vi "Dosing.vi"() -> ()   [LabVIEW 2019]
uses:
  <vilib>/NI/Current Value Table/Type Defs/Single Tag.ctl
  <vilib>/NI/Current Value Table/Type Defs/Data Types.ctl
  <vilib>/NI/STM/TCP/Read Meta Data (TCP Ref).vi
  <vilib>/NI/STM/TCP/Get Connection Reference (TCP).vi
  <vilib>/NI/AMC/Read Termination Message.vi
  <vilib>/NI/AMC/Create Single Message.vi
  <vilib>/NI/AMC/Update Message Routing Info.vi
  <vilib>/NI/STM/TCP/Read Meta Data (TCP Clst).vi
  <vilib>/NI/AMC/Globals.vi
  <vilib>/NI/STM/TCP/Write Message (TCP).vi
  <vilib>/NI/AMC/Send Message.vi
  <vilib>/NI/AMC/AMC.lvlib
  <vilib>/NI/STM/NI STM.lvlib
  <vilib>/NI/Current Value Table/Current Value Table.lvlib
panel:
  in  "Sulfuric Proc 3":dbl=2.0 caption="ml Acid Proc 3" min=0.0 max=5000.0 step=1.0
  in  "Trig Sulfuric Proc 3":bool caption="Trigger Dose"
  in  "Sulfuric Proc 2":dbl=2.0 caption="ml Acid Proc 2" min=0.0 max=5000.0 step=1.0
  in  "Trig Sulfuric Proc 2":bool caption="Trigger Dose"
  in  "Sulfuric Proc 1":dbl=2.0 caption="ml Acid Proc 1" min=0.0 max=5000.0 step=1.0
  in  "Trig Sulfuric Proc1":bool caption="Trigger Dose"
  in  "LEV Proc 3":dbl=2.0 caption="ml Lev Proc 3" min=0.0 max=1000.0 step=1.0
  in  "Trig Level Proc 3":bool caption="Trigger Dose"
  in  "LEV Proc 2":dbl=2.0 caption="ml Lev Proc 2" min=0.0 max=1000.0 step=1.0
  in  "Trig Level Proc 2":bool caption="Trigger Dose"
  in  "LEV Proc 1":dbl=2.0 caption="ml Lev Proc 1" min=0.0 max=1000.0 step=1.0
  in  "Trig Level Proc1":bool caption="Trigger Dose"
  in  "UCON Proc 3":dbl=2.0 caption="ml UCON Proc 3" min=0.0 max=1000.0 step=1.0
  in  "Trig UCON Proc 3":bool caption="Trigger Dose"
  in  "UCON Proc 2":dbl=2.0 caption="ml UCON Proc 2" min=0.0 max=1000.0 step=1.0
  in  "Trig UCON Proc 2":bool caption="Trigger Dose"
  in  "UCON Proc 1":dbl=2.0 caption="ml UCON Proc 1" min=0.0 max=1000.0 step=1.0
  in  "Trig UCON Proc 1":bool caption="Trigger Dose"
  in  "SPS Proc 3":dbl=2.0 caption="ml SPS Proc 3" min=0.0 max=1000.0 step=1.0
  in  "Trig SPS Proc 3":bool caption="Trigger Dose"
  in  "SPS Proc 2":dbl=2.0 caption="ml SPS Proc 2" min=0.0 max=1000.0 step=1.0
  in  "Trig SPS Proc 2":bool caption="Trigger Dose"
  in  "SPS Proc 1":dbl=2.0 caption="ml SPS Proc 1" min=0.0 max=1000.0 step=1.0
  in  "Trig SPS Proc 1":bool caption="Trigger Dose"
  out "Run Enabled":bool
  in  "Dosing":bool
  in  "Mixing Tank":bool
  in  "Process 3":bool
  in  "Process 2":bool
  in  "Process 1":bool
  out "status":string
  in  "Home Btn":bool
  in  "Facilities Btn":bool
  # "SPS"
  # "UCON"
  # "Leveler"
  # "Sulfuric Acid"
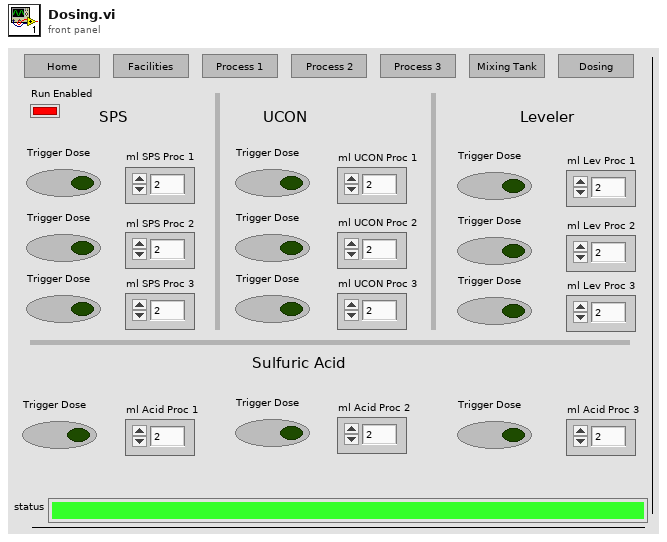
[diagram p1: front panel]
types:
  T1 = typedef "Current Value Table.lvlib/Single Tag.ctl" = cluster{"Data Type":T2, "Name":string, "Value":string, "Description":string}
  T2 = typedef "Current Value Table.lvlib/Data Types.ctl" = enum16{"Double", "Single", "I64", "I32", "I16", "I8", "U64", "U32", "U16", "U8", "String", "Boolean", "Array of U8", "Array of U16", "Array of U32", "Array of U64", "Array of I64", "Array of I32", "Array of I16", "Array of I8", "Array of Double", "Array of Single", "Array of Boolean", "Array of String"}
  T3 = typedef "AMC.lvlib/Message Queue.ctl" = refnum<queue>
  T4 = typedef "NI STM.lvlib/TCP Connection Info.ctl" = cluster{"connection ID":refnum<k5>, "meta data":T5[]}
  T5 = typedef "NI STM.lvlib/MetaDataElement.ctl" = string
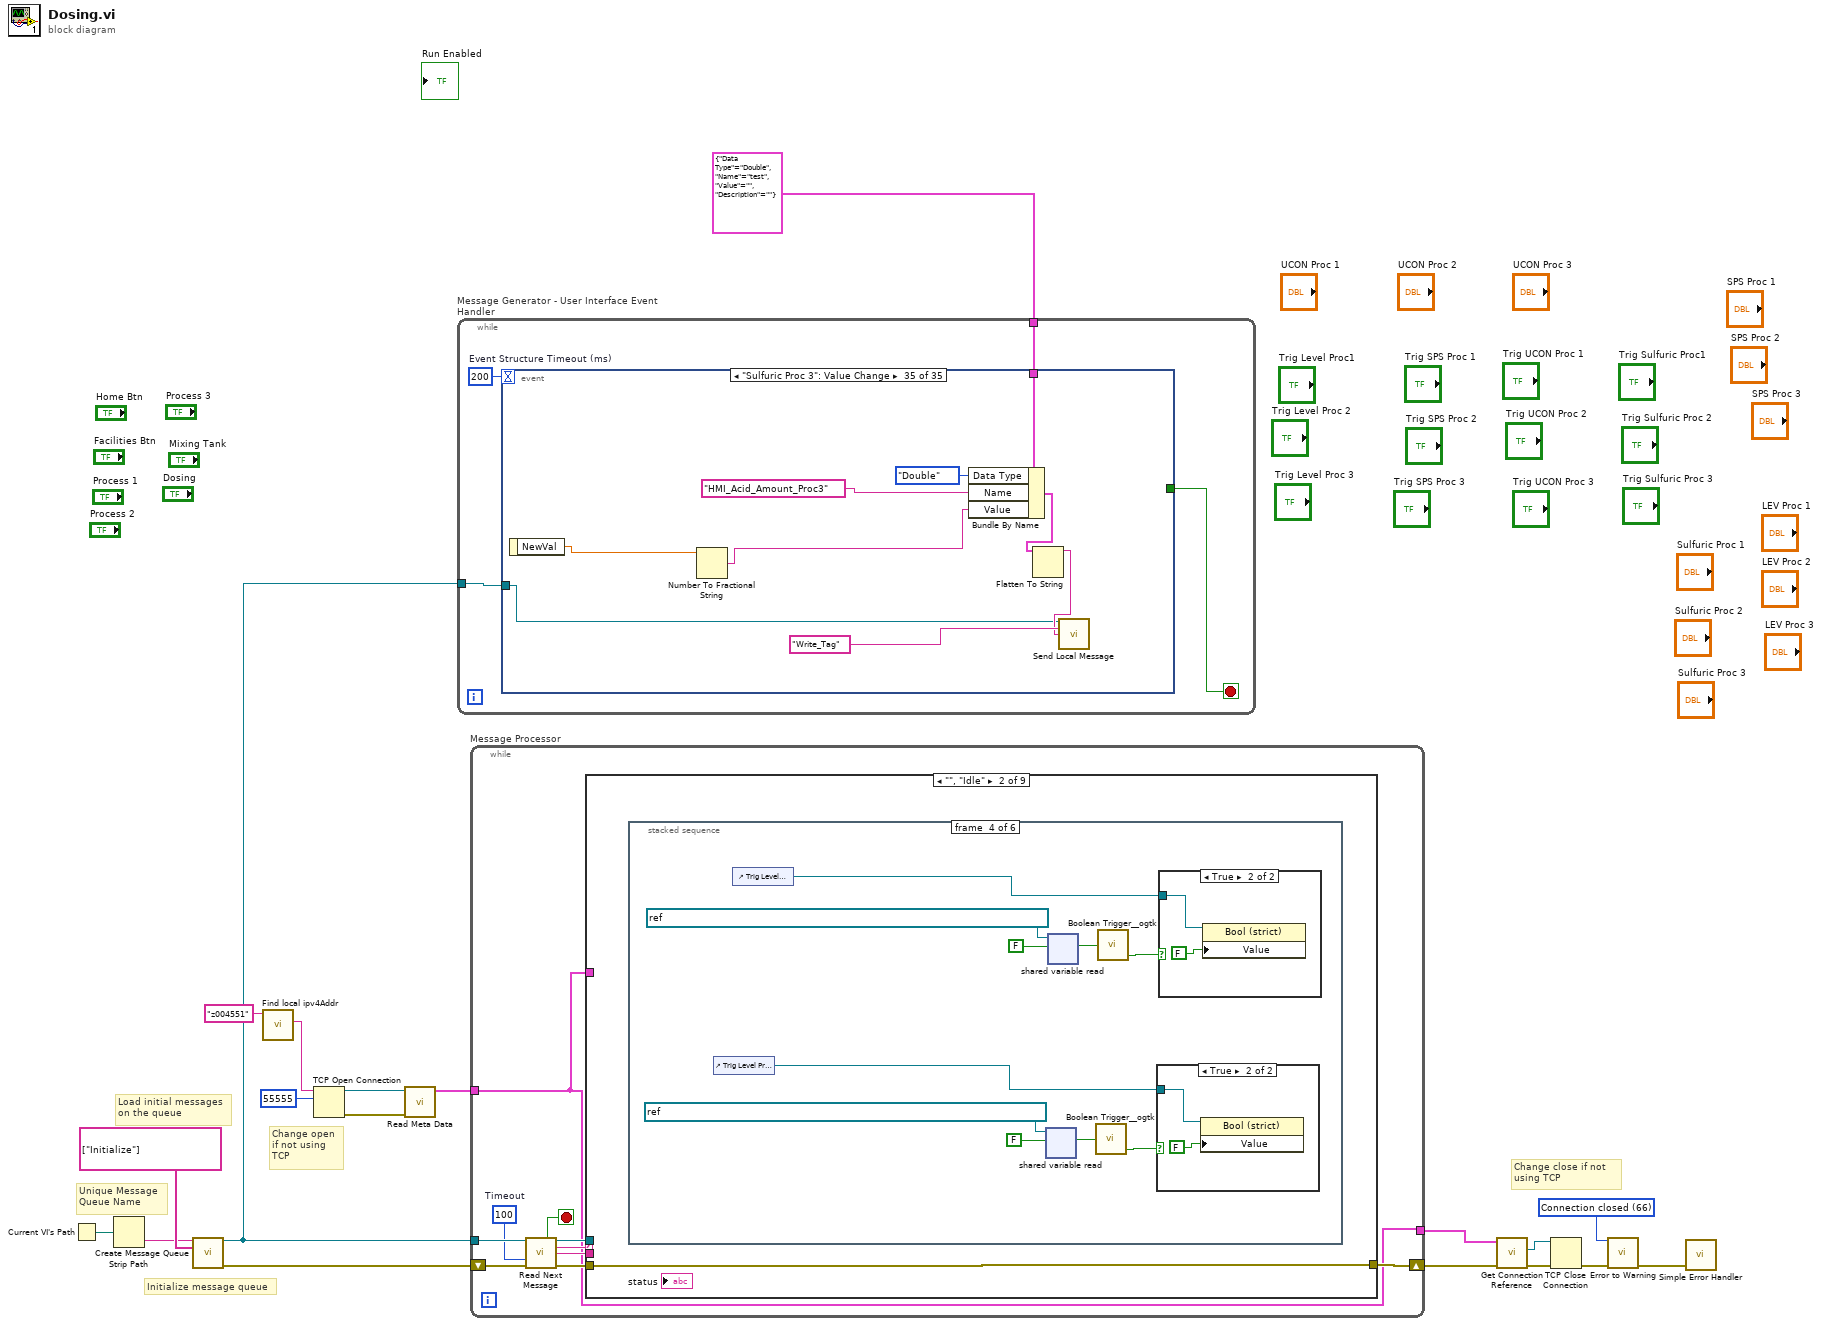
[diagram p0: block diagram]
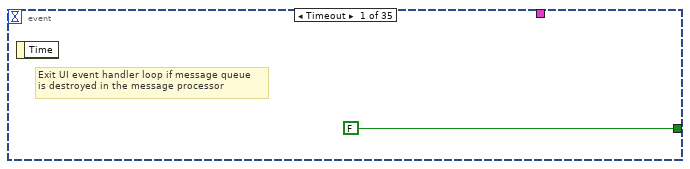
[diagram p2: hidden frame]
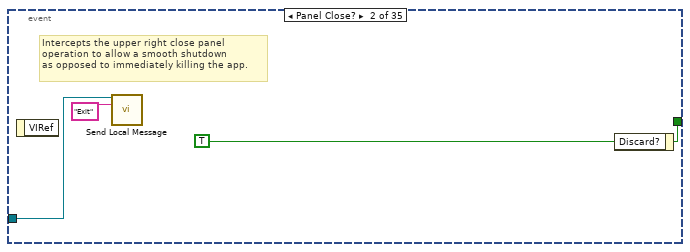
[diagram p3: hidden frame]
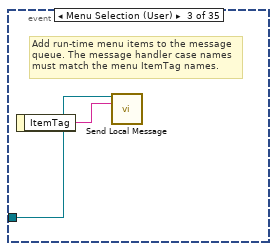
[diagram p4: hidden frame]
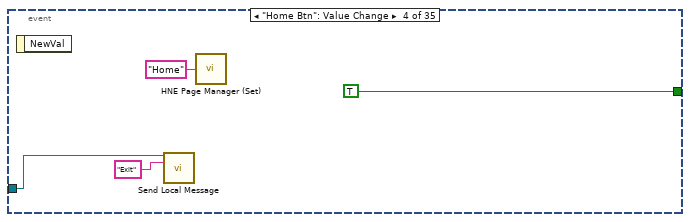
[diagram p5: hidden frame]
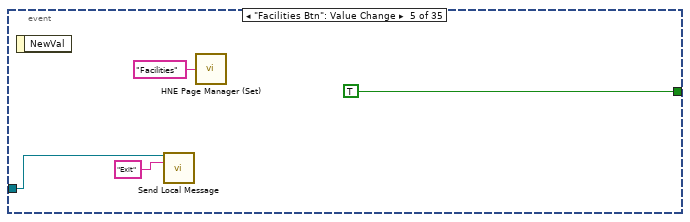
[diagram p6: hidden frame]
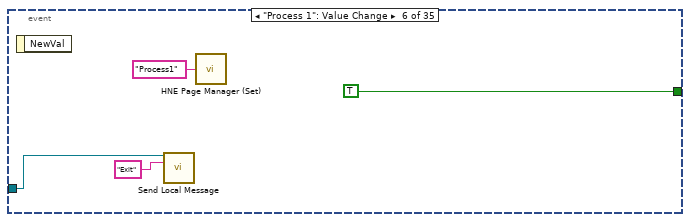
[diagram p7: hidden frame]
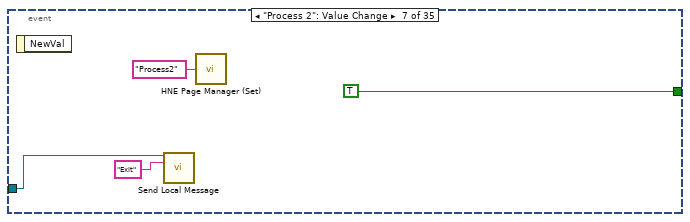
[diagram p8: hidden frame]
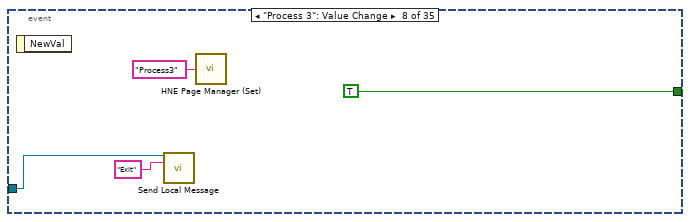
[diagram p9: hidden frame]
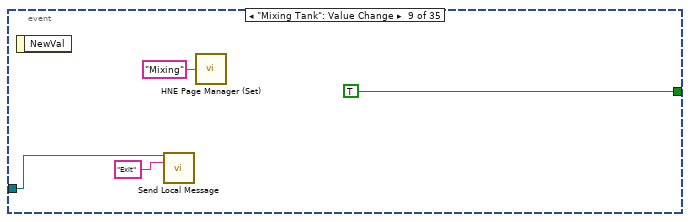
[diagram p10: hidden frame]
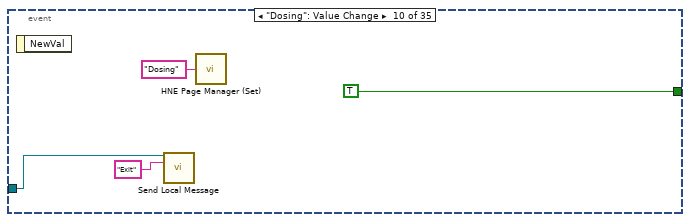
[diagram p11: hidden frame]
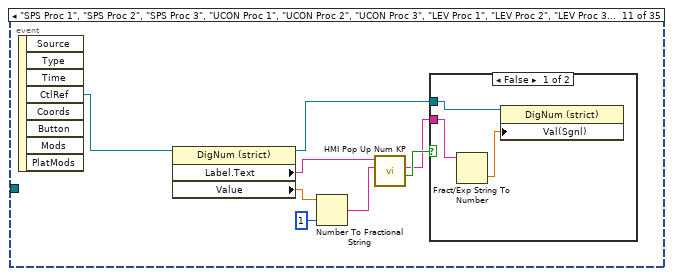
[diagram p12: hidden frame]
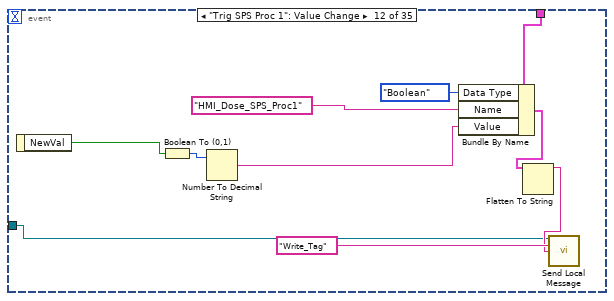
[diagram p14: hidden frame]
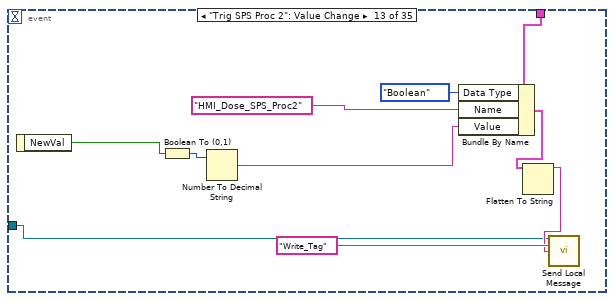
[diagram p15: hidden frame]
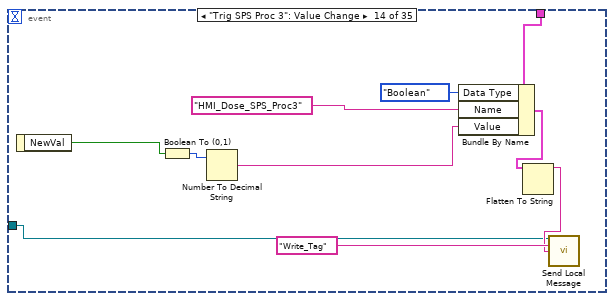
[diagram p16: hidden frame]
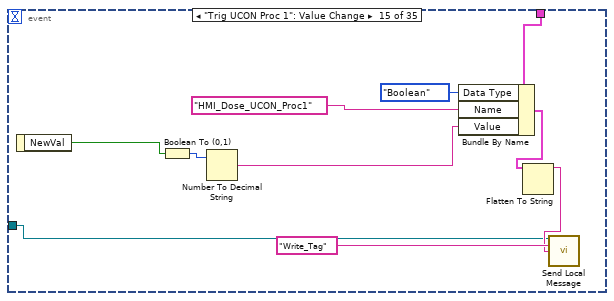
[diagram p17: hidden frame]
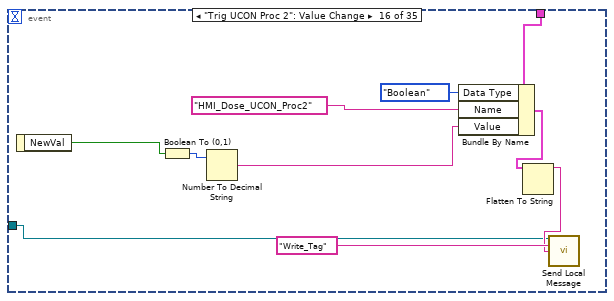
[diagram p18: hidden frame]
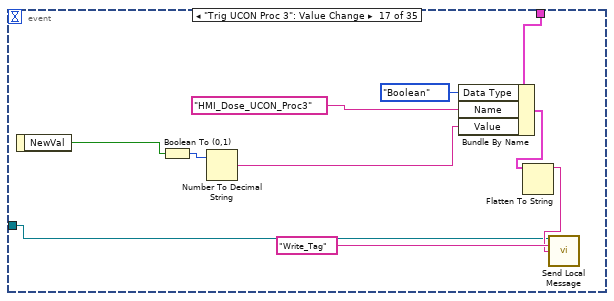
[diagram p19: hidden frame]
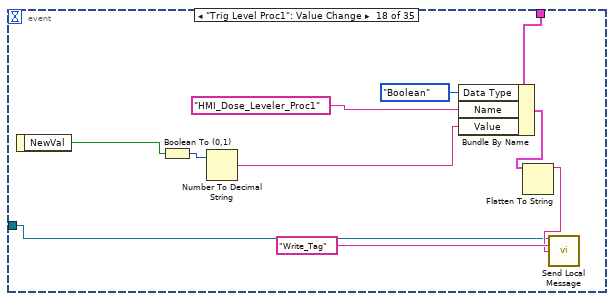
[diagram p20: hidden frame]
diagram:
  w8 = 66 items=["No Error", "Argument Error", "Memory Full", "Out of Zone", "End of File", "File Already Open", "Generic File IO Error", "File Not Found", "File Permission Error", "Disk Full", "Duplicate Path", "Too Many Files Open", "Not Enabled", "Resource File Not Found", "Cannot Add Resource", "Resource Not Found", "Image Not Found", "Image Memory Error", "Pen Does Not Exist", "Config Bad Type", "Config Token Not Found", "Config Parse Error", "Config Memory Error", "Bad External Code Format", "Bad External Code Offset", "External Code Not Present", "Null Window", "Destroy Window Mixup", "Null Menu", "Print Aborted", "Bad Print Record", "Print Driver Error", "Windows Error During Print", "Memory Error During Print", "Print Dialog Error", "Generic Print Error", "Invalid Device Refnum", "Device Not Found", "Device Parameter Error", "Device Unit Error", "Can't Open Device", "Device Call Aborted", "Generic Error", "Cancelled By User", "Object ID Too Low", "Object ID Too High", "Object Not In Heap", "Unknown Heap", "Bad DefProc ID", "DefProc Not In Table", "Message Out Of Range", "Null Method", "Unknown Message", "Manager Call Not Supported", "Bad address", "Connection In progress", "Connection timed out", "Connection is already in progress", "Network attribute not supported", "Network error", "Address in use", "System out of memory", "Connection aborted", "Connection refused", "Connection is not connected", "Connection is already connected", "Connection closed", "Initialize error (interapplication manager)", "Bad occurrence", "Wait on unbound occurrence handler", "Occurrence queue overflow", "Bad path", "Semaphore not signaled", "Unrecognized type (interapplication manager)"] ("1st Error to Convert")
  # "Change close if not using TCP"
  # "Change open if not using TCP"
  # "Initialize message queue"
  # "Unique Message\nQueue Name"
  # "Load initial messages\non the queue"
  n1 = Current VI's Path() -> (path=w15:path)
  n2 = Strip Path(path=w15) -> (name=w18:string)  [unwired: 1 out]
  n3 = call <vilib>:"Create Message Queue.vi"("message queue name"=w18, "initial message names"=string[] ["Initialize"]) -> ("message queue out"=w17:T3, "error out"=w16:errorcluster)  [unwired: 12 in]
  n4 = call "Find local ipv4Addr.vi"("MachineToFind"="z004551") -> ("name"=w11:string)  [unwired: 9 in, 1 out]
  n5 = TCP Open Connection(address=w11, remote port or service name=u16 55555 ("remote port")) -> (connection ID=w13:refnum<k5>, error out=w12:errorcluster)  [unwired: 1 in, 2 out]
  n6 = call-poly <vilib>:"Read Meta Data.vi"("error in"=w12, "connection ID"=w13) -> ("connection info out"=w3:T4)  [unwired: 7 in, 2 out]
  n7 = while "Message Generator - User Interface Event Handler" {
    tunnel: w17 -> [w21]
    tunnel: T1 {"Data Type"=enum."Double", "Name"="test", "Value"="", "Description"=""} ("Tag") -> [w20]
    stop <- w22 stop-if-true
    w23 = 200  # Event Structure Timeout (ms)
    n8 = event shown="[34] \"Sulfuric Proc 3\": Value Change" {
      selector: _ -> [_ _ _ _ _ _ _ _ _ _ _ _ _ _ _ _ _ _ _ _ _ _ _ _ _ _ _ _ _ _ _ _ _ _ _]
      dyn-events: _ -> [_ _ _ _ _ _ _ _ _ _ _ _ _ _ _ _ _ _ _ _ _ _ _ _ _ _ _ _ _ _ _ _ _ _ _]
      timeout: w23 -> [_ _ _ _ _ _ _ _ _ _ _ _ _ _ _ _ _ _ _ _ _ _ _ _ _ _ _ _ _ _ _ _ _ _ _]
      tunnel: [FALSE ("Discard?") w27 _ TRUE ("Discard?") TRUE ("Discard?") TRUE ("Discard?") TRUE ("Discard?") TRUE ("Discard?") TRUE ("Discard?") TRUE ("Discard?") _ _ _ _ _ _ _ _ _ _ _ _ _ _ _ _ _ _ _ _ _ _ _ _ _] -> w22
      tunnel: w21 -> [_ w25 w28 w30 w34 w38 w42 w46 w50 w54 _ w70 w80 w90 w100 w110 w120 w130 w140 w150 w160 w170 w180 w190 w199 w208 w217 w226 w235 w244 w253 w262 w271 w280 w289]
      tunnel: w20 -> [_ _ _ _ _ _ _ _ _ _ _ w69 w79 w89 w99 w109 w119 w129 w139 w149 w159 w169 w179 w189 w198 w207 w216 w225 w234 w243 w252 w261 w270 w279 w288]
      event Timeout {
        # "Exit UI event handler loop if message queue\nis destroyed in the message processor"
        n9 = event-data() -> ()  [unwired: 2 out]
      }
      event Panel Close? {
        w27 = TRUE ("Discard?")
        # "Intercepts the upper right close panel\noperation to allow a smooth shutdown\nas opposed to immediately killing the app."
        n10 = event-data() -> ()  [unwired: 2 out]
        n11 = call <vilib>:"Send Local Message.vi"("message queue in"=w25, "message name"="Exit") -> ()  [unwired: 11 in, 3 out]
        n12 = event-data("Discard?"=w27) -> ()  [unwired: 1 in, 1 out]
      }
      event Menu Selection (User) {
        # "Add run-time menu items to the message\nqueue. The message handler case names must match the menu ItemTag names."
        n13 = event-data() -> ("ItemTag"=w29:string)  [unwired: 1 out]
        n14 = call <vilib>:"Send Local Message.vi"("message queue in"=w28, "message name"=w29) -> ()  [unwired: 11 in, 3 out]
      }
      event "Home Btn": Value Change {
        n15 = event-data() -> ()  [unwired: 2 out]
        n16 = call <vilib>:"Send Local Message.vi"("message queue in"=w30, "message name"="Exit") -> ()  [unwired: 11 in, 3 out]
        n17 = call <userlib>:"HNE Page Manager (Set).vi"("Next Page"="Home") -> ()  [unwired: 4 in, 1 out]
      }
      event "Facilities Btn": Value Change {
        n18 = event-data() -> ()  [unwired: 2 out]
        n19 = call <vilib>:"Send Local Message.vi"("message queue in"=w34, "message name"="Exit") -> ()  [unwired: 11 in, 3 out]
        n20 = call <userlib>:"HNE Page Manager (Set).vi"("Next Page"="Facilities") -> ()  [unwired: 4 in, 1 out]
      }
      event "Process 1": Value Change {
        n21 = event-data() -> ()  [unwired: 2 out]
        n22 = call <vilib>:"Send Local Message.vi"("message queue in"=w38, "message name"="Exit") -> ()  [unwired: 11 in, 3 out]
        n23 = call <userlib>:"HNE Page Manager (Set).vi"("Next Page"="Process1") -> ()  [unwired: 4 in, 1 out]
      }
      event "Process 2": Value Change {
        n24 = event-data() -> ()  [unwired: 2 out]
        n25 = call <vilib>:"Send Local Message.vi"("message queue in"=w42, "message name"="Exit") -> ()  [unwired: 11 in, 3 out]
        n26 = call <userlib>:"HNE Page Manager (Set).vi"("Next Page"="Process2") -> ()  [unwired: 4 in, 1 out]
      }
      event "Process 3": Value Change {
        n27 = event-data() -> ()  [unwired: 2 out]
        n28 = call <vilib>:"Send Local Message.vi"("message queue in"=w46, "message name"="Exit") -> ()  [unwired: 11 in, 3 out]
        n29 = call <userlib>:"HNE Page Manager (Set).vi"("Next Page"="Process3") -> ()  [unwired: 4 in, 1 out]
      }
      event "Mixing Tank": Value Change {
        n30 = event-data() -> ()  [unwired: 2 out]
        n31 = call <vilib>:"Send Local Message.vi"("message queue in"=w50, "message name"="Exit") -> ()  [unwired: 11 in, 3 out]
        n32 = call <userlib>:"HNE Page Manager (Set).vi"("Next Page"="Mixing") -> ()  [unwired: 4 in, 1 out]
      }
      event "Dosing": Value Change {
        n33 = event-data() -> ()  [unwired: 2 out]
        n34 = call <vilib>:"Send Local Message.vi"("message queue in"=w54, "message name"="Exit") -> ()  [unwired: 11 in, 3 out]
        n35 = call <userlib>:"HNE Page Manager (Set).vi"("Next Page"="Dosing") -> ()  [unwired: 4 in, 1 out]
      }
      event "SPS Proc 1", "SPS Proc 2", "SPS Proc 3", "UCON Proc 1", "UCON Proc 2", "UCON Proc 3", "LEV Proc 1", "LEV Proc 2", "LEV Proc 3", "Sulfuric Proc 1", "Sulfuric Proc 2", "Sulfuric Proc 3": Mouse Up {
        n36 = event-data() -> ("CtlRef"=w58:refnum<vi>)  [unwired: 8 out]
        n37 = property class="DigNum (strict)"(reference=w58) -> (reference out=w59:refnum<vi>, "Label.Text"=w65:string, "Value"=w64:dbl)  [unwired: 1 in, 1 out]
        n38 = Number To Fractional String(number=w64, precision (6)=i16 1) -> (F-format string=w63:string)  [unwired: 2 in]
        n39 = call <userlib>:"HMI Pop Up Num KP.vi"("String In"=w63, "Message In"=w65) -> ("Canceled"=w61:bool, "String Out"=w60:string)  [unwired: 8 in]
        n40 = case shown="False" w61 {
          tunnel: w60 -> [w67 _]
          tunnel: w59 -> [w68 _]
          frame False {
            n41 = Fract/Exp String To Number(string=w67) -> (number=w66:dbl)  [unwired: 3 in, 1 out]
            n42 = property class="DigNum (strict)"(reference=w68, "Val(Sgnl)"=w66) -> ()  [unwired: 1 in, 2 out]
          }
          frame True {
          }
        }
      }
      event "Trig SPS Proc 1": Value Change {
        n43 = event-data() -> ("NewVal"=w71:bool)  [unwired: 1 out]
        n44 = Boolean To (0,1)(Boolean=w71) -> (0, 1=w78:i16)
        n45 = Number To Decimal String(number=w78) -> (decimal integer string=w75:string)  [unwired: 1 in]
        n46 = Bundle By Name(cluster=w69, "Data Type"=Data_Types."Boolean", "Name"="HMI_Dose_SPS_Proc1", "Value"=w75) -> (w74:T1)
        n47 = Flatten To String(anything=w74) -> (data string=w72:string)  [unwired: 3 in, 2 out]
        n48 = call <vilib>:"Send Local Message.vi"("message queue in"=w70, "message name"="Write_Tag", "message value"=w72) -> ()  [unwired: 10 in, 3 out]
      }
      event "Trig SPS Proc 2": Value Change {
        n49 = event-data() -> ("NewVal"=w81:bool)  [unwired: 1 out]
        n50 = Boolean To (0,1)(Boolean=w81) -> (0, 1=w88:i16)
        n51 = Number To Decimal String(number=w88) -> (decimal integer string=w85:string)  [unwired: 1 in]
        n52 = Bundle By Name(cluster=w79, "Data Type"=Data_Types."Boolean", "Name"="HMI_Dose_SPS_Proc2", "Value"=w85) -> (w84:T1)
        n53 = Flatten To String(anything=w84) -> (data string=w82:string)  [unwired: 3 in, 2 out]
        n54 = call <vilib>:"Send Local Message.vi"("message queue in"=w80, "message name"="Write_Tag", "message value"=w82) -> ()  [unwired: 10 in, 3 out]
      }
      event "Trig SPS Proc 3": Value Change {
        n55 = event-data() -> ("NewVal"=w91:bool)  [unwired: 1 out]
        n56 = Boolean To (0,1)(Boolean=w91) -> (0, 1=w98:i16)
        n57 = Number To Decimal String(number=w98) -> (decimal integer string=w95:string)  [unwired: 1 in]
        n58 = Bundle By Name(cluster=w89, "Data Type"=Data_Types."Boolean", "Name"="HMI_Dose_SPS_Proc3", "Value"=w95) -> (w94:T1)
        n59 = Flatten To String(anything=w94) -> (data string=w92:string)  [unwired: 3 in, 2 out]
        n60 = call <vilib>:"Send Local Message.vi"("message queue in"=w90, "message name"="Write_Tag", "message value"=w92) -> ()  [unwired: 10 in, 3 out]
      }
      event "Trig UCON Proc 1": Value Change {
        n61 = event-data() -> ("NewVal"=w101:bool)  [unwired: 1 out]
        n62 = Boolean To (0,1)(Boolean=w101) -> (0, 1=w108:i16)
        n63 = Number To Decimal String(number=w108) -> (decimal integer string=w105:string)  [unwired: 1 in]
        n64 = Bundle By Name(cluster=w99, "Data Type"=Data_Types."Boolean", "Name"="HMI_Dose_UCON_Proc1", "Value"=w105) -> (w104:T1)
        n65 = Flatten To String(anything=w104) -> (data string=w102:string)  [unwired: 3 in, 2 out]
        n66 = call <vilib>:"Send Local Message.vi"("message queue in"=w100, "message name"="Write_Tag", "message value"=w102) -> ()  [unwired: 10 in, 3 out]
      }
      event "Trig UCON Proc 2": Value Change {
        n67 = event-data() -> ("NewVal"=w111:bool)  [unwired: 1 out]
        n68 = Boolean To (0,1)(Boolean=w111) -> (0, 1=w118:i16)
        n69 = Number To Decimal String(number=w118) -> (decimal integer string=w115:string)  [unwired: 1 in]
        n70 = Bundle By Name(cluster=w109, "Data Type"=Data_Types."Boolean", "Name"="HMI_Dose_UCON_Proc2", "Value"=w115) -> (w114:T1)
        n71 = Flatten To String(anything=w114) -> (data string=w112:string)  [unwired: 3 in, 2 out]
        n72 = call <vilib>:"Send Local Message.vi"("message queue in"=w110, "message name"="Write_Tag", "message value"=w112) -> ()  [unwired: 10 in, 3 out]
      }
      event "Trig UCON Proc 3": Value Change {
        n73 = event-data() -> ("NewVal"=w121:bool)  [unwired: 1 out]
        n74 = Boolean To (0,1)(Boolean=w121) -> (0, 1=w128:i16)
        n75 = Number To Decimal String(number=w128) -> (decimal integer string=w125:string)  [unwired: 1 in]
        n76 = Bundle By Name(cluster=w119, "Data Type"=Data_Types."Boolean", "Name"="HMI_Dose_UCON_Proc3", "Value"=w125) -> (w124:T1)
        n77 = Flatten To String(anything=w124) -> (data string=w122:string)  [unwired: 3 in, 2 out]
        n78 = call <vilib>:"Send Local Message.vi"("message queue in"=w120, "message name"="Write_Tag", "message value"=w122) -> ()  [unwired: 10 in, 3 out]
      }
      event "Trig Level Proc1": Value Change {
        n79 = event-data() -> ("NewVal"=w131:bool)  [unwired: 1 out]
        n80 = Boolean To (0,1)(Boolean=w131) -> (0, 1=w138:i16)
        n81 = Number To Decimal String(number=w138) -> (decimal integer string=w135:string)  [unwired: 1 in]
        n82 = Bundle By Name(cluster=w129, "Data Type"=Data_Types."Boolean", "Name"="HMI_Dose_Leveler_Proc1", "Value"=w135) -> (w134:T1)
        n83 = Flatten To String(anything=w134) -> (data string=w132:string)  [unwired: 3 in, 2 out]
        n84 = call <vilib>:"Send Local Message.vi"("message queue in"=w130, "message name"="Write_Tag", "message value"=w132) -> ()  [unwired: 10 in, 3 out]
      }
      event "Trig Level Proc 2": Value Change {
        n85 = event-data() -> ("NewVal"=w141:bool)  [unwired: 1 out]
        n86 = Boolean To (0,1)(Boolean=w141) -> (0, 1=w148:i16)
        n87 = Number To Decimal String(number=w148) -> (decimal integer string=w145:string)  [unwired: 1 in]
        n88 = Bundle By Name(cluster=w139, "Data Type"=Data_Types."Boolean", "Name"="HMI_Dose_Leveler_Proc2", "Value"=w145) -> (w144:T1)
        n89 = Flatten To String(anything=w144) -> (data string=w142:string)  [unwired: 3 in, 2 out]
        n90 = call <vilib>:"Send Local Message.vi"("message queue in"=w140, "message name"="Write_Tag", "message value"=w142) -> ()  [unwired: 10 in, 3 out]
      }
      event "Trig Level Proc 3": Value Change {
        n91 = event-data() -> ("NewVal"=w151:bool)  [unwired: 1 out]
        n92 = Boolean To (0,1)(Boolean=w151) -> (0, 1=w158:i16)
        n93 = Number To Decimal String(number=w158) -> (decimal integer string=w155:string)  [unwired: 1 in]
        n94 = Bundle By Name(cluster=w149, "Data Type"=Data_Types."Boolean", "Name"="HMI_Dose_Leveler_Proc3", "Value"=w155) -> (w154:T1)
        n95 = Flatten To String(anything=w154) -> (data string=w152:string)  [unwired: 3 in, 2 out]
        n96 = call <vilib>:"Send Local Message.vi"("message queue in"=w150, "message name"="Write_Tag", "message value"=w152) -> ()  [unwired: 10 in, 3 out]
      }
      event "Trig Sulfuric Proc1": Value Change {
        n97 = event-data() -> ("NewVal"=w161:bool)  [unwired: 1 out]
        n98 = Boolean To (0,1)(Boolean=w161) -> (0, 1=w168:i16)
        n99 = Number To Decimal String(number=w168) -> (decimal integer string=w165:string)  [unwired: 1 in]
        n100 = Bundle By Name(cluster=w159, "Data Type"=Data_Types."Boolean", "Name"="HMI_Dose_Acid_Proc1", "Value"=w165) -> (w164:T1)
        n101 = Flatten To String(anything=w164) -> (data string=w162:string)  [unwired: 3 in, 2 out]
        n102 = call <vilib>:"Send Local Message.vi"("message queue in"=w160, "message name"="Write_Tag", "message value"=w162) -> ()  [unwired: 10 in, 3 out]
      }
      event "Trig Sulfuric Proc 2": Value Change {
        n103 = event-data() -> ("NewVal"=w171:bool)  [unwired: 1 out]
        n104 = Boolean To (0,1)(Boolean=w171) -> (0, 1=w178:i16)
        n105 = Number To Decimal String(number=w178) -> (decimal integer string=w175:string)  [unwired: 1 in]
        n106 = Bundle By Name(cluster=w169, "Data Type"=Data_Types."Boolean", "Name"="HMI_Dose_Acid_Proc2", "Value"=w175) -> (w174:T1)
        n107 = Flatten To String(anything=w174) -> (data string=w172:string)  [unwired: 3 in, 2 out]
        n108 = call <vilib>:"Send Local Message.vi"("message queue in"=w170, "message name"="Write_Tag", "message value"=w172) -> ()  [unwired: 10 in, 3 out]
      }
      event "Trig Sulfuric Proc 3": Value Change {
        n109 = event-data() -> ("NewVal"=w181:bool)  [unwired: 1 out]
        n110 = Boolean To (0,1)(Boolean=w181) -> (0, 1=w188:i16)
        n111 = Number To Decimal String(number=w188) -> (decimal integer string=w185:string)  [unwired: 1 in]
        n112 = Bundle By Name(cluster=w179, "Data Type"=Data_Types."Boolean", "Name"="HMI_Dose_Acid_Proc3", "Value"=w185) -> (w184:T1)
        n113 = Flatten To String(anything=w184) -> (data string=w182:string)  [unwired: 3 in, 2 out]
        n114 = call <vilib>:"Send Local Message.vi"("message queue in"=w180, "message name"="Write_Tag", "message value"=w182) -> ()  [unwired: 10 in, 3 out]
      }
      event "SPS Proc 1": Value Change {
        n115 = event-data() -> ("NewVal"=w191:dbl)  [unwired: 1 out]
        n116 = Number To Fractional String(number=w191) -> (F-format string=w192:string)  [unwired: 3 in]
        n117 = Bundle By Name(cluster=w189, "Data Type"=Data_Types."Double", "Name"="HMI_SPS_Amount_Proc1", "Value"=w192) -> (w195:T1)
        n118 = Flatten To String(anything=w195) -> (data string=w193:string)  [unwired: 3 in, 2 out]
        n119 = call <vilib>:"Send Local Message.vi"("message queue in"=w190, "message name"="Write_Tag", "message value"=w193) -> ()  [unwired: 10 in, 3 out]
      }
      event "SPS Proc 2": Value Change {
        n120 = event-data() -> ("NewVal"=w200:dbl)  [unwired: 1 out]
        n121 = Number To Fractional String(number=w200) -> (F-format string=w201:string)  [unwired: 3 in]
        n122 = Bundle By Name(cluster=w198, "Data Type"=Data_Types."Double", "Name"="HMI_SPS_Amount_Proc2", "Value"=w201) -> (w204:T1)
        n123 = Flatten To String(anything=w204) -> (data string=w202:string)  [unwired: 3 in, 2 out]
        n124 = call <vilib>:"Send Local Message.vi"("message queue in"=w199, "message name"="Write_Tag", "message value"=w202) -> ()  [unwired: 10 in, 3 out]
      }
      event "SPS Proc 3": Value Change {
        n125 = event-data() -> ("NewVal"=w209:dbl)  [unwired: 1 out]
        n126 = Number To Fractional String(number=w209) -> (F-format string=w210:string)  [unwired: 3 in]
        n127 = Bundle By Name(cluster=w207, "Data Type"=Data_Types."Double", "Name"="HMI_SPS_Amount_Proc3", "Value"=w210) -> (w213:T1)
        n128 = Flatten To String(anything=w213) -> (data string=w211:string)  [unwired: 3 in, 2 out]
        n129 = call <vilib>:"Send Local Message.vi"("message queue in"=w208, "message name"="Write_Tag", "message value"=w211) -> ()  [unwired: 10 in, 3 out]
      }
      event "UCON Proc 1": Value Change {
        n130 = event-data() -> ("NewVal"=w218:dbl)  [unwired: 1 out]
        n131 = Number To Fractional String(number=w218) -> (F-format string=w219:string)  [unwired: 3 in]
        n132 = Bundle By Name(cluster=w216, "Data Type"=Data_Types."Double", "Name"="HMI_UCON_Amount_Proc1", "Value"=w219) -> (w222:T1)
        n133 = Flatten To String(anything=w222) -> (data string=w220:string)  [unwired: 3 in, 2 out]
        n134 = call <vilib>:"Send Local Message.vi"("message queue in"=w217, "message name"="Write_Tag", "message value"=w220) -> ()  [unwired: 10 in, 3 out]
      }
      event "UCON Proc 2": Value Change {
        n135 = event-data() -> ("NewVal"=w227:dbl)  [unwired: 1 out]
        n136 = Number To Fractional String(number=w227) -> (F-format string=w228:string)  [unwired: 3 in]
        n137 = Bundle By Name(cluster=w225, "Data Type"=Data_Types."Double", "Name"="HMI_UCON_Amount_Proc2", "Value"=w228) -> (w231:T1)
        n138 = Flatten To String(anything=w231) -> (data string=w229:string)  [unwired: 3 in, 2 out]
        n139 = call <vilib>:"Send Local Message.vi"("message queue in"=w226, "message name"="Write_Tag", "message value"=w229) -> ()  [unwired: 10 in, 3 out]
      }
      event "UCON Proc 3": Value Change {
        n140 = event-data() -> ("NewVal"=w236:dbl)  [unwired: 1 out]
        n141 = Number To Fractional String(number=w236) -> (F-format string=w237:string)  [unwired: 3 in]
        n142 = Bundle By Name(cluster=w234, "Data Type"=Data_Types."Double", "Name"="HMI_UCON_Amount_Proc3", "Value"=w237) -> (w240:T1)
        n143 = Flatten To String(anything=w240) -> (data string=w238:string)  [unwired: 3 in, 2 out]
        n144 = call <vilib>:"Send Local Message.vi"("message queue in"=w235, "message name"="Write_Tag", "message value"=w238) -> ()  [unwired: 10 in, 3 out]
      }
      event "LEV Proc 1": Value Change {
        n145 = event-data() -> ("NewVal"=w245:dbl)  [unwired: 1 out]
        n146 = Number To Fractional String(number=w245) -> (F-format string=w246:string)  [unwired: 3 in]
        n147 = Bundle By Name(cluster=w243, "Data Type"=Data_Types."Double", "Name"="HMI_Leveler_Amount_Proc1", "Value"=w246) -> (w249:T1)
        n148 = Flatten To String(anything=w249) -> (data string=w247:string)  [unwired: 3 in, 2 out]
        n149 = call <vilib>:"Send Local Message.vi"("message queue in"=w244, "message name"="Write_Tag", "message value"=w247) -> ()  [unwired: 10 in, 3 out]
      }
      event "LEV Proc 2": Value Change {
        n150 = event-data() -> ("NewVal"=w254:dbl)  [unwired: 1 out]
        n151 = Number To Fractional String(number=w254) -> (F-format string=w255:string)  [unwired: 3 in]
        n152 = Bundle By Name(cluster=w252, "Data Type"=Data_Types."Double", "Name"="HMI_Leveler_Amount_Proc2", "Value"=w255) -> (w258:T1)
        n153 = Flatten To String(anything=w258) -> (data string=w256:string)  [unwired: 3 in, 2 out]
        n154 = call <vilib>:"Send Local Message.vi"("message queue in"=w253, "message name"="Write_Tag", "message value"=w256) -> ()  [unwired: 10 in, 3 out]
      }
      event "LEV Proc 3": Value Change {
        n155 = event-data() -> ("NewVal"=w263:dbl)  [unwired: 1 out]
        n156 = Number To Fractional String(number=w263) -> (F-format string=w264:string)  [unwired: 3 in]
        n157 = Bundle By Name(cluster=w261, "Data Type"=Data_Types."Double", "Name"="HMI_Leveler_Amount_Proc3", "Value"=w264) -> (w267:T1)
        n158 = Flatten To String(anything=w267) -> (data string=w265:string)  [unwired: 3 in, 2 out]
        n159 = call <vilib>:"Send Local Message.vi"("message queue in"=w262, "message name"="Write_Tag", "message value"=w265) -> ()  [unwired: 10 in, 3 out]
      }
      event "Sulfuric Proc 1": Value Change {
        n160 = event-data() -> ("NewVal"=w272:dbl)  [unwired: 1 out]
        n161 = Number To Fractional String(number=w272) -> (F-format string=w273:string)  [unwired: 3 in]
        n162 = Bundle By Name(cluster=w270, "Data Type"=Data_Types."Double", "Name"="HMI_Acid_Amount_Proc1", "Value"=w273) -> (w276:T1)
        n163 = Flatten To String(anything=w276) -> (data string=w274:string)  [unwired: 3 in, 2 out]
        n164 = call <vilib>:"Send Local Message.vi"("message queue in"=w271, "message name"="Write_Tag", "message value"=w274) -> ()  [unwired: 10 in, 3 out]
      }
      event "Sulfuric Proc 2": Value Change {
        n165 = event-data() -> ("NewVal"=w281:dbl)  [unwired: 1 out]
        n166 = Number To Fractional String(number=w281) -> (F-format string=w282:string)  [unwired: 3 in]
        n167 = Bundle By Name(cluster=w279, "Data Type"=Data_Types."Double", "Name"="HMI_Acid_Amount_Proc2", "Value"=w282) -> (w285:T1)
        n168 = Flatten To String(anything=w285) -> (data string=w283:string)  [unwired: 3 in, 2 out]
        n169 = call <vilib>:"Send Local Message.vi"("message queue in"=w280, "message name"="Write_Tag", "message value"=w283) -> ()  [unwired: 10 in, 3 out]
      }
      event "Sulfuric Proc 3": Value Change {
        n170 = event-data() -> ("NewVal"=w290:dbl)  [unwired: 1 out]
        n171 = Number To Fractional String(number=w290) -> (F-format string=w291:string)  [unwired: 3 in]
        n172 = Bundle By Name(cluster=w288, "Data Type"=Data_Types."Double", "Name"="HMI_Acid_Amount_Proc3", "Value"=w291) -> (w294:T1)
        n173 = Flatten To String(anything=w294) -> (data string=w292:string)  [unwired: 3 in, 2 out]
        n174 = call <vilib>:"Send Local Message.vi"("message queue in"=w289, "message name"="Write_Tag", "message value"=w292) -> ()  [unwired: 10 in, 3 out]
      }
    }
  }
  n175 = while "Message Processor" {
    shift-left: w16 -> [w302]
    shift-right: [w306] -> w4
    tunnel: w17 -> [w303]
    tunnel: [w297] -> w2
    tunnel: w3 -> [w297]
    stop <- w305 stop-if-true
    w298 = 100  # Timeout
    n176 = call <vilib>:"Read Next Message.vi"("message queue in"=w303, "timeout (1 ms)"=w298, "error in"=w302) -> ("exit process?"=w305:bool, "message queue out"=w304:T3, "message name"=w300:string, "message value"=w299:string, "error out"=w301:errorcluster)  [unwired: 5 in, 3 out]
    n177 = case shown="\"\", \"Idle\"" w300 {
      selector: w300 -> [_ _ w394 _ _ _ _ _ _]
      tunnel: w304 -> [_ _ _ _ _ _ w473 _ _]
      tunnel: w301 -> [w307 w308 w395 w396 w398 w399 w474 w476 w478]
      tunnel: [w307 w308 w395 errorcluster {"status"=FALSE, "code"=0, "source"=""} ("error out") w398 w399 w472 w476 w477] -> w306
      tunnel: w299 -> [_ _ _ _ _ _ _ _ w479]
      tunnel: w297 -> [_ _ _ _ _ _ _ _ w480]
      frame "---------- Framework Operations ----------" {
        # "Dummy case to add a seperator in the Case Structure menu"
      }
      frame "", "Idle" {
        n178 = stacked-sequence {
          frame #0 {
            n179 = control-ref of="Trig SPS Proc 2"() -> (w310:refnum<vi>)
            n180 = shared-variable-read(refnum<k21> "ni.var.psp://z004551/CDL0100 ReadWriteTags/HMI_Dose_SPS_Proc1" ("shared variable refnum in"), FALSE) -> (w315:bool)  [unwired: 1 in, 3 out]
            n181 = shared-variable-read(refnum<k21> "ni.var.psp://z004551/CDL0100 ReadWriteTags/HMI_Dose_SPS_Proc2" ("shared variable refnum in"), FALSE) -> (w311:bool)  [unwired: 1 in, 3 out]
            n182 = call <userlib>:"Boolean Trigger__ogtk.vi"("Boolean Input"=w315) -> ("Falling Edge"=w314:bool)  [unwired: 1 in, 1 out]
            n183 = call <userlib>:"Boolean Trigger__ogtk.vi"("Boolean Input"=w311) -> ("Falling Edge"=w309:bool)  [unwired: 1 in, 1 out]
            n184 = case shown="True" w314 {
              frame False {
              }
              frame True {
                n185 = local write "Trig SPS Proc 1"(FALSE) -> ()
              }
            }
            n186 = case shown="True" w309 {
              tunnel: w310 -> [_ w319]
              frame False {
              }
              frame True {
                n187 = property class="Bool (strict)"(reference=w319, "Value"=FALSE) -> ()  [unwired: 1 in, 2 out]
              }
            }
          }
          frame #1 {
            n188 = control-ref of="Trig SPS Proc 3"() -> (w326:refnum<vi>)
            n189 = control-ref of="Trig UCON Proc 1"() -> (w321:refnum<vi>)
            n190 = shared-variable-read(refnum<k21> "ni.var.psp://z004551/CDL0100 ReadWriteTags/HMI_Dose_SPS_Proc3" ("shared variable refnum in"), FALSE) -> (w328:bool)  [unwired: 1 in, 3 out]
            n191 = shared-variable-read(refnum<k21> "ni.var.psp://z004551/CDL0100 ReadWriteTags/HMI_Dose_UCON_Proc1" ("shared variable refnum in"), FALSE) -> (w323:bool)  [unwired: 1 in, 3 out]
            n192 = call <userlib>:"Boolean Trigger__ogtk.vi"("Boolean Input"=w328) -> ("Falling Edge"=w327:bool)  [unwired: 1 in, 1 out]
            n193 = call <userlib>:"Boolean Trigger__ogtk.vi"("Boolean Input"=w323) -> ("Falling Edge"=w322:bool)  [unwired: 1 in, 1 out]
            n194 = case shown="True" w327 {
              tunnel: w326 -> [_ w334]
              frame False {
              }
              frame True {
                n195 = property class="Bool (strict)"(reference=w334, "Value"=FALSE) -> ()  [unwired: 1 in, 2 out]
              }
            }
            n196 = case shown="True" w322 {
              tunnel: w321 -> [_ w332]
              frame False {
              }
              frame True {
                n197 = property class="Bool (strict)"(reference=w332, "Value"=FALSE) -> ()  [unwired: 1 in, 2 out]
              }
            }
          }
          frame #2 {
            n198 = control-ref of="Trig UCON Proc 3"() -> (w335:refnum<vi>)
            n199 = control-ref of="Trig UCON Proc 2"() -> (w340:refnum<vi>)
            n200 = shared-variable-read(refnum<k21> "ni.var.psp://z004551/CDL0100 ReadWriteTags/HMI_Dose_UCON_Proc2" ("shared variable refnum in"), FALSE) -> (w342:bool)  [unwired: 1 in, 3 out]
            n201 = shared-variable-read(refnum<k21> "ni.var.psp://z004551/CDL0100 ReadWriteTags/HMI_Dose_UCON_Proc3" ("shared variable refnum in"), FALSE) -> (w337:bool)  [unwired: 1 in, 3 out]
            n202 = call <userlib>:"Boolean Trigger__ogtk.vi"("Boolean Input"=w342) -> ("Falling Edge"=w341:bool)  [unwired: 1 in, 1 out]
            n203 = call <userlib>:"Boolean Trigger__ogtk.vi"("Boolean Input"=w337) -> ("Falling Edge"=w336:bool)  [unwired: 1 in, 1 out]
            n204 = case shown="True" w341 {
              tunnel: w340 -> [_ w348]
              frame False {
              }
              frame True {
                n205 = property class="Bool (strict)"(reference=w348, "Value"=FALSE) -> ()  [unwired: 1 in, 2 out]
              }
            }
            n206 = case shown="True" w336 {
              tunnel: w335 -> [_ w346]
              frame False {
              }
              frame True {
                n207 = property class="Bool (strict)"(reference=w346, "Value"=FALSE) -> ()  [unwired: 1 in, 2 out]
              }
            }
          }
          frame #3 {
            n208 = control-ref of="Trig Level Proc 2"() -> (w349:refnum<vi>)
            n209 = control-ref of="Trig Level Proc1"() -> (w354:refnum<vi>)
            n210 = shared-variable-read(refnum<k21> "ni.var.psp://z004551/CDL0100 ReadWriteTags/HMI_Dose_Leveler_Proc2" ("shared variable refnum in"), FALSE) -> (w351:bool)  [unwired: 1 in, 3 out]
            n211 = shared-variable-read(refnum<k21> "ni.var.psp://z004551/CDL0100 ReadWriteTags/HMI_Dose_Leveler_Proc1" ("shared variable refnum in"), FALSE) -> (w356:bool)  [unwired: 1 in, 3 out]
            n212 = call <userlib>:"Boolean Trigger__ogtk.vi"("Boolean Input"=w351) -> ("Falling Edge"=w350:bool)  [unwired: 1 in, 1 out]
            n213 = call <userlib>:"Boolean Trigger__ogtk.vi"("Boolean Input"=w356) -> ("Falling Edge"=w355:bool)  [unwired: 1 in, 1 out]
            n214 = case shown="True" w350 {
              tunnel: w349 -> [_ w360]
              frame False {
              }
              frame True {
                n215 = property class="Bool (strict)"(reference=w360, "Value"=FALSE) -> ()  [unwired: 1 in, 2 out]
              }
            }
            n216 = case shown="True" w355 {
              tunnel: w354 -> [_ w362]
              frame False {
              }
              frame True {
                n217 = property class="Bool (strict)"(reference=w362, "Value"=FALSE) -> ()  [unwired: 1 in, 2 out]
              }
            }
          }
          frame #4 {
            n218 = control-ref of="Trig Sulfuric Proc1"() -> (w363:refnum<vi>)
            n219 = control-ref of="Trig Level Proc 3"() -> (w368:refnum<vi>)
            n220 = shared-variable-read(refnum<k21> "ni.var.psp://z004551/CDL0100 ReadWriteTags/HMI_Dose_Leveler_Proc3" ("shared variable refnum in"), FALSE) -> (w370:bool)  [unwired: 1 in, 3 out]
            n221 = shared-variable-read(refnum<k21> "ni.var.psp://z004551/CDL0100 ReadWriteTags/HMI_Dose_Acid_Proc1" ("shared variable refnum in"), FALSE) -> (w365:bool)  [unwired: 1 in, 3 out]
            n222 = call <userlib>:"Boolean Trigger__ogtk.vi"("Boolean Input"=w370) -> ("Falling Edge"=w369:bool)  [unwired: 1 in, 1 out]
            n223 = call <userlib>:"Boolean Trigger__ogtk.vi"("Boolean Input"=w365) -> ("Falling Edge"=w364:bool)  [unwired: 1 in, 1 out]
            n224 = case shown="True" w369 {
              tunnel: w368 -> [_ w376]
              frame False {
              }
              frame True {
                n225 = property class="Bool (strict)"(reference=w376, "Value"=FALSE) -> ()  [unwired: 1 in, 2 out]
              }
            }
            n226 = case shown="True" w364 {
              tunnel: w363 -> [_ w374]
              frame False {
              }
              frame True {
                n227 = property class="Bool (strict)"(reference=w374, "Value"=FALSE) -> ()  [unwired: 1 in, 2 out]
              }
            }
          }
          frame #5 {
            n228 = control-ref of="Trig Sulfuric Proc 3"() -> (w378:refnum<vi>)
            n229 = control-ref of="Trig Sulfuric Proc 2"() -> (w383:refnum<vi>)
            n230 = control-ref of="status"() -> (w377:refnum<vi>)
            n231 = call <userlib>:"TAE Format Alarm Ticker.vi"("Alarm Ticker Ref"=w377) -> ()  [unwired: 15 in]
            n232 = shared-variable-read(refnum<k21> "ni.var.psp://z004551/CDL0100 ReadWriteTags/HMI_Dose_Acid_Proc2" ("shared variable refnum in"), FALSE) -> (w385:bool)  [unwired: 1 in, 3 out]
            n233 = shared-variable-read(refnum<k21> "ni.var.psp://z004551/CDL0100 ReadWriteTags/HMI_Dose_Acid_Proc3" ("shared variable refnum in"), FALSE) -> (w380:bool)  [unwired: 1 in, 3 out]
            n234 = call <userlib>:"Boolean Trigger__ogtk.vi"("Boolean Input"=w385) -> ("Falling Edge"=w384:bool)  [unwired: 1 in, 1 out]
            n235 = call <userlib>:"Boolean Trigger__ogtk.vi"("Boolean Input"=w380) -> ("Falling Edge"=w379:bool)  [unwired: 1 in, 1 out]
            n236 = case shown="True" w384 {
              tunnel: w383 -> [_ w391]
              frame False {
              }
              frame True {
                n237 = property class="Bool (strict)"(reference=w391, "Value"=FALSE) -> ()  [unwired: 1 in, 2 out]
              }
            }
            n238 = case shown="True" w379 {
              tunnel: w378 -> [_ w389]
              frame False {
              }
              frame True {
                n239 = property class="Bool (strict)"(reference=w389, "Value"=FALSE) -> ()  [unwired: 1 in, 2 out]
              }
            }
          }
        }
      }
      frame "Missing Message Handler", Default {
        # "Call this case if a message is received that is not handled \nby any other case. Typically this is a programming error\nas a result of a typo or unhandled message/missing message handler."
        n240 = Format Into String(format string="DevError: Missing message handler for '%s\" message." ("message"), w394) -> (resulting string=w392:string)  [unwired: 2 in, 1 out]
        n241 = One Button Dialog(message=w392) -> ()  [unwired: 2 out]
      }
      frame "Error" {
        # "General Error Case - this case is called if an error is passed using the error cluster below. Typically most new errors should be handed in each individual case and not passed in the rror cluster. If necessary a custom error handler case should be added and called from other cases."
        n242 = call <vilib>:"Simple Error Handler.vi"("error in (no error)"=w396) -> ()  [unwired: 1 in, 8 out]
      }
      frame "---------- Generic Operations ----------" {
        # "Dummy case to add a seperator in the Case Structure menu"
      }
      frame "Initialize" {
        # "Initialize the state variables and user interface"
        n243 = stacked-sequence {
          frame #0 {
            n244 = shared-variable-read(refnum<k21> "ni.var.psp://z004551/CDL0100 ReadWriteTags/HMI_Dose_SPS_Proc2" ("shared variable refnum in"), FALSE) -> (w401:bool)  [unwired: 1 in, 3 out]
            n245 = shared-variable-read(refnum<k21> "ni.var.psp://z004551/CDL0100 ReadWriteTags/HMI_Dose_SPS_Proc1" ("shared variable refnum in"), FALSE) -> (w409:bool)  [unwired: 1 in, 3 out]
            n246 = shared-variable-read(refnum<k21> "ni.var.psp://z004551/CDL0100 ReadWriteTags/HMI_SPS_Amount_Proc2" ("shared variable refnum in"), 0.0) -> (w400:dbl)  [unwired: 1 in, 3 out]
            n247 = shared-variable-read(refnum<k21> "ni.var.psp://z004551/CDL0100 ReadWriteTags/HMI_SPS_Amount_Proc1" ("shared variable refnum in"), 0.0) -> (w406:dbl)  [unwired: 1 in, 3 out]
            n248 = local write "Trig SPS Proc 2"(w401) -> ()
            n249 = local write "Trig SPS Proc 1"(w409) -> ()
            n250 = local write "SPS Proc 2"(w400) -> ()
            n251 = local write "SPS Proc 1"(w406) -> ()
          }
          frame #1 {
            n252 = shared-variable-read(refnum<k21> "ni.var.psp://z004551/CDL0100 ReadWriteTags/HMI_SPS_Amount_Proc3" ("shared variable refnum in"), 0.0) -> (w418:dbl)  [unwired: 1 in, 3 out]
            n253 = shared-variable-read(refnum<k21> "ni.var.psp://z004551/CDL0100 ReadWriteTags/HMI_Dose_SPS_Proc3" ("shared variable refnum in"), FALSE) -> (w419:bool)  [unwired: 1 in, 3 out]
            n254 = shared-variable-read(refnum<k21> "ni.var.psp://z004551/CDL0100 ReadWriteTags/HMI_UCON_Amount_Proc1" ("shared variable refnum in"), 0.0) -> (w412:dbl)  [unwired: 1 in, 3 out]
            n255 = shared-variable-read(refnum<k21> "ni.var.psp://z004551/CDL0100 ReadWriteTags/HMI_Dose_UCON_Proc1" ("shared variable refnum in"), FALSE) -> (w413:bool)  [unwired: 1 in, 3 out]
            n256 = local write "Trig UCON Proc 1"(w413) -> ()
            n257 = local write "UCON Proc 1"(w412) -> ()
            n258 = local write "Trig SPS Proc 3"(w419) -> ()
            n259 = local write "SPS Proc 3"(w418) -> ()
          }
          frame #2 {
            n260 = shared-variable-read(refnum<k21> "ni.var.psp://z004551/CDL0100 ReadWriteTags/HMI_UCON_Amount_Proc3" ("shared variable refnum in"), 0.0) -> (w424:dbl)  [unwired: 1 in, 3 out]
            n261 = shared-variable-read(refnum<k21> "ni.var.psp://z004551/CDL0100 ReadWriteTags/HMI_Dose_UCON_Proc3" ("shared variable refnum in"), FALSE) -> (w425:bool)  [unwired: 1 in, 3 out]
            n262 = shared-variable-read(refnum<k21> "ni.var.psp://z004551/CDL0100 ReadWriteTags/HMI_UCON_Amount_Proc2" ("shared variable refnum in"), 0.0) -> (w431:dbl)  [unwired: 1 in, 3 out]
            n263 = shared-variable-read(refnum<k21> "ni.var.psp://z004551/CDL0100 ReadWriteTags/HMI_Dose_UCON_Proc2" ("shared variable refnum in"), FALSE) -> (w430:bool)  [unwired: 1 in, 3 out]
            n264 = local write "UCON Proc 3"(w424) -> ()
            n265 = local write "UCON Proc 2"(w431) -> ()
            n266 = local write "Trig UCON Proc 3"(w425) -> ()
            n267 = local write "Trig UCON Proc 2"(w430) -> ()
          }
          frame #3 {
            n268 = shared-variable-read(refnum<k21> "ni.var.psp://z004551/CDL0100 ReadWriteTags/HMI_Leveler_Amount_Proc1" ("shared variable refnum in"), 0.0) -> (w442:dbl)  [unwired: 1 in, 3 out]
            n269 = shared-variable-read(refnum<k21> "ni.var.psp://z004551/CDL0100 ReadWriteTags/HMI_Leveler_Amount_Proc2" ("shared variable refnum in"), 0.0) -> (w436:dbl)  [unwired: 1 in, 3 out]
            n270 = shared-variable-read(refnum<k21> "ni.var.psp://z004551/CDL0100 ReadWriteTags/HMI_Dose_Leveler_Proc1" ("shared variable refnum in"), FALSE) -> (w443:bool)  [unwired: 1 in, 3 out]
            n271 = shared-variable-read(refnum<k21> "ni.var.psp://z004551/CDL0100 ReadWriteTags/HMI_Dose_Leveler_Proc2" ("shared variable refnum in"), FALSE) -> (w437:bool)  [unwired: 1 in, 3 out]
            n272 = local write "LEV Proc 2"(w436) -> ()
            n273 = local write "Trig Level Proc 2"(w437) -> ()
            n274 = local write "Trig Level Proc1"(w443) -> ()
            n275 = local write "LEV Proc 1"(w442) -> ()
          }
          frame #4 {
            n276 = shared-variable-read(refnum<k21> "ni.var.psp://z004551/CDL0100 ReadWriteTags/HMI_Leveler_Amount_Proc3" ("shared variable refnum in"), 0.0) -> (w454:dbl)  [unwired: 1 in, 3 out]
            n277 = shared-variable-read(refnum<k21> "ni.var.psp://z004551/CDL0100 ReadWriteTags/HMI_Dose_Leveler_Proc3" ("shared variable refnum in"), FALSE) -> (w455:bool)  [unwired: 1 in, 3 out]
            n278 = shared-variable-read(refnum<k21> "ni.var.psp://z004551/CDL0100 ReadWriteTags/HMI_Acid_Amount_Proc1" ("shared variable refnum in"), 0.0) -> (w448:dbl)  [unwired: 1 in, 3 out]
            n279 = shared-variable-read(refnum<k21> "ni.var.psp://z004551/CDL0100 ReadWriteTags/HMI_Dose_Acid_Proc1" ("shared variable refnum in"), FALSE) -> (w449:bool)  [unwired: 1 in, 3 out]
            n280 = local write "Trig Sulfuric Proc1"(w449) -> ()
            n281 = local write "LEV Proc 3"(w454) -> ()
            n282 = local write "Trig Level Proc 3"(w455) -> ()
            n283 = local write "Sulfuric Proc 1"(w448) -> ()
          }
          frame #5 {
            n284 = shared-variable-read(refnum<k21> "ni.var.psp://z004551/CDL0100 ReadWriteTags/HMI_Acid_Amount_Proc3" ("shared variable refnum in"), 0.0) -> (w460:dbl)  [unwired: 1 in, 3 out]
            n285 = shared-variable-read(refnum<k21> "ni.var.psp://z004551/CDL0100 ReadWriteTags/HMI_Dose_Acid_Proc3" ("shared variable refnum in"), FALSE) -> (w461:bool)  [unwired: 1 in, 3 out]
            n286 = shared-variable-read(refnum<k21> "ni.var.psp://z004551/CDL0100 ReadWriteTags/HMI_Acid_Amount_Proc2" ("shared variable refnum in"), 0.0) -> (w466:dbl)  [unwired: 1 in, 3 out]
            n287 = shared-variable-read(refnum<k21> "ni.var.psp://z004551/CDL0100 ReadWriteTags/HMI_Dose_Acid_Proc2" ("shared variable refnum in"), FALSE) -> (w467:bool)  [unwired: 1 in, 3 out]
            n288 = local write "Trig Sulfuric Proc 3"(w461) -> ()
            n289 = local write "Sulfuric Proc 3"(w460) -> ()
            n290 = local write "Sulfuric Proc 2"(w466) -> ()
            n291 = local write "Trig Sulfuric Proc 2"(w467) -> ()
          }
        }
      }
      frame "Exit" {
        # "Destroy message queue >> this will halt the UI event handler loop"
        # "Stop the VI\n>> Perform any cleanup tasks in this message case.\n>> Clear display before closing."
        n292 = call <vilib>:"Destroy Message Queue.vi"("message queue in"=w473, "error in"=w474) -> ("error out"=w472:errorcluster)  [unwired: 11 in, 2 out]
        n293 = local write "status"("" ("Status")) -> ()
      }
      frame "---------- Application Operations ----------" {
        # "Dummy case to add a seperator in the Case Structure menu"
      }
      frame "Write_Tag" {
        n294 = call-poly <vilib>:"Write Message.vi"("error in"=w478, "data"=w479, "name"="WriteTag", "connection info in"=w480) -> ("error out"=w477:errorcluster)  [unwired: 6 in, 1 out]
      }
    }
  }
  n295 = call-poly <vilib>:"Get Connection Reference.vi"("error in"=w4, "connection info in"=w2) -> ("error out"=w7:errorcluster, "connection ID out"=w6:refnum<k5>)  [unwired: 8 out]
  n296 = TCP Close Connection(connection ID=w6, error in (no error)=w7) -> (error out=w9:errorcluster)  [unwired: 2 out]
  n297 = call <vilib>:"Error to Warning.vi"("1st Error to Convert"=w8, "error in"=w9) -> ("warning out"=w5:errorcluster)  [unwired: 3 in, 10 out]
  n298 = call <vilib>:"Simple Error Handler.vi"("error in (no error)"=w5) -> ()  [unwired: 4 in, 5 out]
